vi "decode_ext_signals.vi"(0 "VISA resource name":refnum<visa-resource-name>, 2 "previous_status cmd string":string, 5 "analog inputs":dbl[](array[numeric]) format="%#_6p", 7 "COM response delay":u32, 9 "commit?":bool, 11 "error in (no error)":errorcluster) -> (1 "update of COM error status":bool, 3 "excitation filter":u16, 4 "VISA resource name out":refnum<visa-resource-name>, 6 "disk position":bool, 8 "update need commit?":bool, 10 "disk spinning":bool, 12 "dichroic mirror":u16, 13 "emission filter":u16, 14 "cmd string":string, 15 "error out":errorcluster)   [LabVIEW 2016]
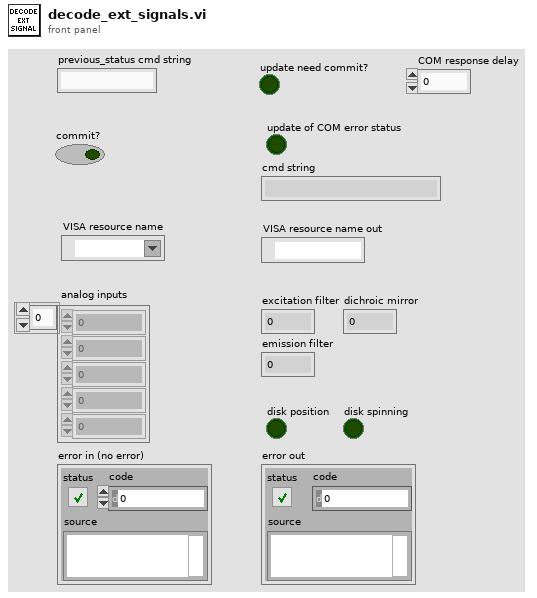
[diagram p1: front panel]
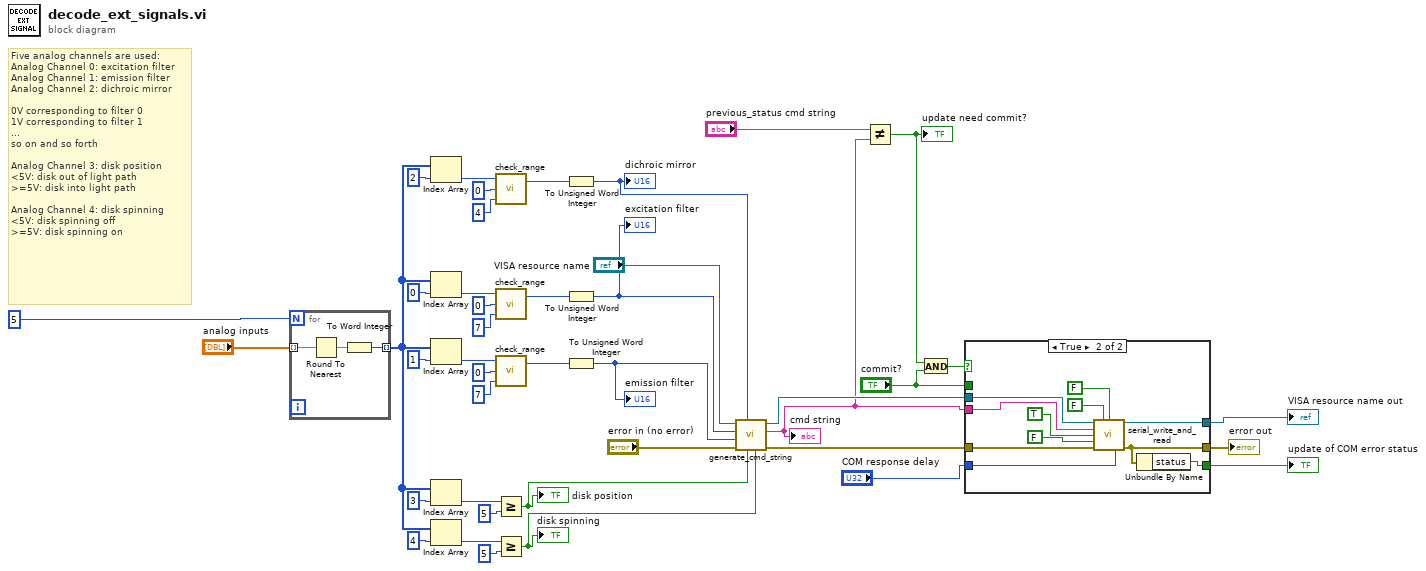
[diagram p0: block diagram]
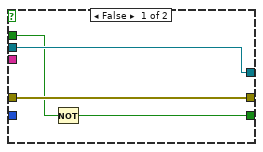
[diagram p2: hidden frame]
diagram:
  # "Five analog channels are used:\nAnalog Channel 0: excitation filter\nAnalog Channel 1: emission filter\nAnalog Channel 2: dichroic mirror\n\n0V corresponding to filter 0\n1V corresponding to filter 1\n...\nso on and so forth\n\nAnalog Channel 3: disk position\n<5V: disk out of light path\n>=5V: disk into light path\n\nAnalog Channel 4: disk spinning\n<5V: disk spinning off\n>=5V: disk spinning on"
  n1 = for {
    N: 5 -> [_]
    tunnel: "analog inputs" -> [w43] mode=indexing
    tunnel: [w44] -> w23 mode=indexing
    n2 = Round To Nearest(number=w43) -> (nearest integer value=w45:dbl)
    n3 = To Word Integer(number=w45) -> (16bit integer=w44:i16)
  }
  n4 = Index Array(array=w23, index=2) -> (element=w26:i16)
  n5 = Index Array(array=w23, index=0) -> (element=w36:i16)
  n6 = Index Array(array=w23, index=1) -> (element=w30:i16)
  n7 = Index Array(array=w23, index=3) -> (element=w19:i16)
  n8 = Index Array(array=w23, index=4) -> (element=w22:i16)
  n9 = call "check_range.vi"("max"=i16 4, "min"=i16 0, "x"=w26) -> ("checked x"=w25:i16)  [unwired: 1 in]
  n10 = call "check_range.vi"("max"=i16 7, "min"=i16 0, "x"=w36) -> ("checked x"=w33:i16)  [unwired: 1 in]
  n11 = call "check_range.vi"("max"=i16 7, "min"=i16 0, "x"=w30) -> ("checked x"=w29:i16)  [unwired: 1 in]
  n12 = Greater Or Equal?(x=w19, y=i16 5) -> (x >= y?=w8:bool)
  "disk position" <- w8
  n13 = Greater Or Equal?(x=w22, y=i16 5) -> (x >= y?=w7:bool)
  "disk spinning" <- w7
  n14 = To Unsigned Word Integer(number=w25) -> (unsigned 16bit integer=w9:u16)
  "dichroic mirror" <- w9
  n15 = To Unsigned Word Integer(number=w33) -> (unsigned 16bit integer=w11:u16)
  "excitation filter" <- w11
  n16 = To Unsigned Word Integer(number=w29) -> (unsigned 16bit integer=w10:u16)
  "emission filter" <- w10
  n17 = call "generate_cmd_string.vi"("disk spinning"=w7, "disk position"=w8, "dichroic mirror"=w9, "error in (no error)"="error in (no error)", "emission filter"=w10, "excitation filter"=w11, "port in"="VISA resource name") -> ("error out"=w13:errorcluster, "cmd string"=w5:string, "port out"=w12:refnum<visa-resource-name>)  [unwired: 2 in]
  "cmd string" <- w5
  n18 = Not Equal?(x="previous_status cmd string", y=w5) -> (x != y?=w2:bool)
  "update need commit?" <- w2
  n19 = And(x=w2, y="commit?") -> (x .and. y?=w4:bool)
  n20 = case shown="True" w4 {
    tunnel: w12 -> [w49 w60]
    tunnel: w13 -> [w48 w59]
    tunnel: [w48 w52] -> w18
    tunnel: [w49 w58] -> w17
    tunnel: w5 -> [_ w53]
    tunnel: [w47 w51] -> w16
    tunnel: "COM response delay" -> [_ w50]
    tunnel: "commit?" -> [w46 _]
    frame False {
      n21 = Not(x=w46) -> (.not. x?=w47:bool)
    }
    frame True {
      n22 = call "serial_write_and_read.vi"("port name in"=w60, "reconnect?"=FALSE, "disconnect?"=FALSE, "write buffer"=w53, "do writing?"=TRUE, "expecting response?"=FALSE, "error in"=w59, "COM response delay"=w50) -> ("port name out"=w58:refnum<visa-resource-name>, "error out"=w52:errorcluster)  [unwired: 5 in, 1 out]
      n23 = Unbundle By Name(w52) -> ("status"=w51:bool)
    }
  }
  "VISA resource name out" <- w17
  "error out" <- w18
  "update of COM error status" <- w16
